vi "Get JSON.vi"(11 "ConfigFromJSON in":refnum<class "Config from JSON.lvclass">) -> (2 "<JSON>":string, 3 "ConfigFromJSON out":refnum<class "Config from JSON.lvclass">)   [LabVIEW 2024, in "Config from JSON.lvclass"]
uses:
  Config from JSON.lvclass
  Config from JSON.lvclass/Config from JSON.ctl
  <vilib>/JDP Science/JSONtext/Config Files/Config File.lvclass/Config File.ctl
  <vilib>/JDP Science/JSONtext/Config Files/Config File.lvclass
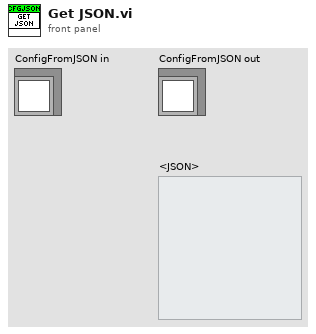
[diagram p1: front panel]
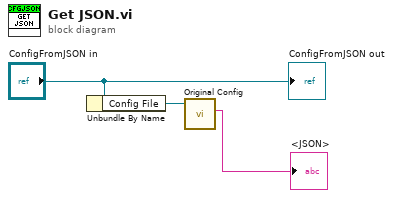
[diagram p0: block diagram]
diagram:
  n1 = Unbundle By Name("ConfigFromJSON in") -> ("Config File"=w1:refnum<class "Config File.lvclass">)
  n2 = call <vilib>:"Original Config.vi"("Config File in"=w1) -> ("Original Config (as read from the file)"=→"<JSON>":string)  [unwired: 10 in]
  "ConfigFromJSON out" <- "ConfigFromJSON in"
